vi "Read Surge Drop Parameters.vi"(0 "VISA resource name":refnum<visa-resource-name>, 11 "error in (no error)":errorcluster) -> (4 "VISA resource name out":refnum<visa-resource-name>, 6 "Surge Drop Voltage (V)":dbl, 8 "Surge Drop Start Time (ms)":dbl, 10 "Surge Drop Duration (ms)":dbl, 15 "error out":errorcluster)   [LabVIEW 2016, in "APT 300XAC Series.lvlib"]
doc: "Reads the surge drop parameters from the power source instrument.\n\nNote :\nProgram Mode : Step Parameter (Can be configured in every step individually).\nManual Mode : System Parameter ( Change in mode affect all steps and memory)\nDC Mode : Not Supported"
uses:
  APT 300XAC Series.lvlib
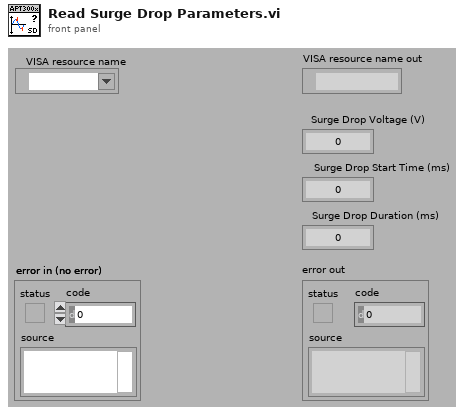
[diagram p1: front panel]
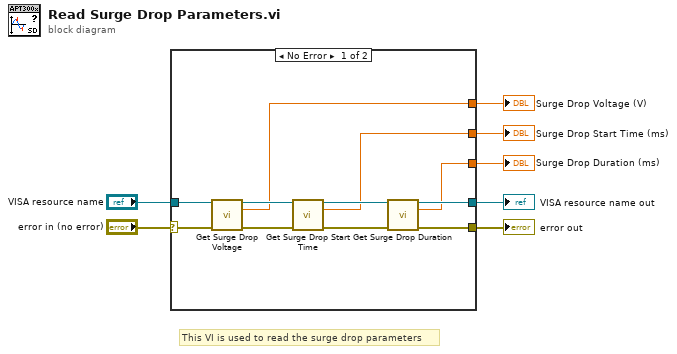
[diagram p0: block diagram]
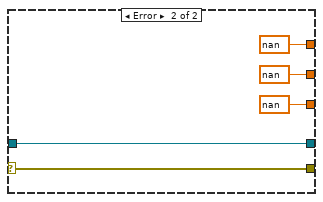
[diagram p2: hidden frame]
diagram:
  # "This VI is used to read the surge drop parameters"
  n1 = case shown="No Error" "error in (no error)" {
    selector: "error in (no error)" -> [w17 w22]
    tunnel: [w12 w22] -> w6
    tunnel: [w11 w23] -> w5
    tunnel: "VISA resource name" -> [w18 w23]
    tunnel: [w10 nan ("Surge Drop Duration")] -> w3
    tunnel: [w9 nan ("Surge Drop Location")] -> w2
    tunnel: [w8 nan ("Surge Drop Voltage")] -> w1
    frame No Error {
      n2 = call "Get Surge Drop Voltage.vi"("VISA resource name"=w18, "error in (no error)"=w17) -> ("VISA resource name out"=w15:refnum<visa-resource-name>, "Surge Drop Voltage (V)"=w8:dbl, "error out"=w16:errorcluster)  [unwired: 11 in]
      n3 = call "Get Surge Drop Start Time.vi"("VISA resource name"=w15, "error in (no error)"=w16) -> ("VISA resource name out"=w14:refnum<visa-resource-name>, "Surge Drop Start Time (ms)"=w9:dbl, "error out"=w13:errorcluster)  [unwired: 11 in]
      n4 = call "Get Surge Drop Duration.vi"("VISA resource name"=w14, "error in (no error)"=w13) -> ("VISA resource name out"=w11:refnum<visa-resource-name>, "Surge Drop Duration (ms)"=w10:dbl, "error out"=w12:errorcluster)  [unwired: 11 in]
    }
    frame Error {
    }
  }
  "error out" <- w6
  "VISA resource name out" <- w5
  "Surge Drop Duration (ms)" <- w3
  "Surge Drop Start Time (ms)" <- w2
  "Surge Drop Voltage (V)" <- w1
